vi "ReadWrite.ProcessData.Commit.vi"(8 "error in":errorcluster, 11 "ReadWrite in":refnum<class "ReadWrite.lvclass">) -> (0 "error out":errorcluster, 3 "ReadWrite out":refnum<class "ReadWrite.lvclass">)   [LabVIEW 2024, in "VS Plugin Data Access Engine.lvlib" / "ReadWrite.lvclass"]
uses:
  ReadWrite.lvclass
  ReadWrite.lvclass/ReadWrite.ctl
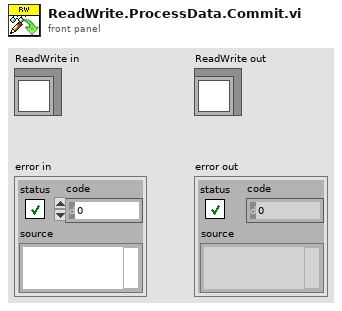
[diagram p1: front panel]
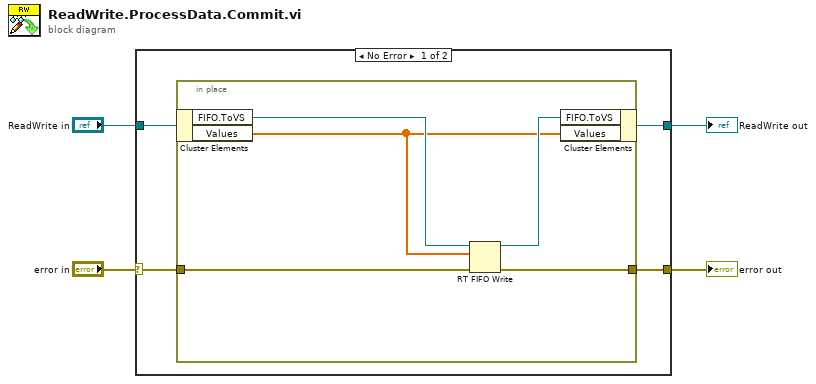
[diagram p0: block diagram]
diagram:
  n1 = case shown="No Error" "error in" {
    selector: "error in" -> [w8 w15]
    tunnel: [w7 w15] -> w3
    tunnel: [w5 w14] -> w1
    tunnel: "ReadWrite in" -> [w6 w14]
    frame No Error {
      n2 = in-place {
        in-place-border: w8 -> [w12]
        in-place-border: [w13] -> w7
        n3 = in-place-cluster #1(w6) -> ("FIFO.ToVS"=w11:refnum<k33>, "Values"=w9:dbl[])
        n4 = RT FIFO Write(0:w11, 1:w9, 3:w12) -> (8:w10:refnum<k33>, 11:w13:errorcluster)  [unwired: 2 in, 2 out]
        n5 = in-place-cluster #1("FIFO.ToVS"=w10, "Values"=w9) -> (w5:refnum<class "ReadWrite.lvclass">)
      }
    }
    frame Error {
    }
  }
  "error out" <- w3
  "ReadWrite out" <- w1
